vi "niRFUtil MT UTIL GenerateFilterCoefficients.vi"(9 "interpolation factor":i32=128, 10 "# of zero crossings":i32=16) -> (0 "full array size":i32, 1 "Differences (scaled)":T1 min=0 max=127 format="%.2f", 2 "Filter Coefficients (scaled)":T1 min=0 max=127 format="%.2f", 3 "Filter Coefficients (unscaled)":T1 min=0 max=127 format="%.2f")   [LabVIEW 2015, in "niRFUtil.lvlib"]
uses:
  niRFUtil.lvlib
  Includes/niRFUtil INC Real Array.ctl
  <vilib>/Analysis/4window.llb/windowTd.ctl
  <vilib>/Analysis/NI_AALBase.lvlib
  <vilib>/Analysis/NI_AALPro.lvlib
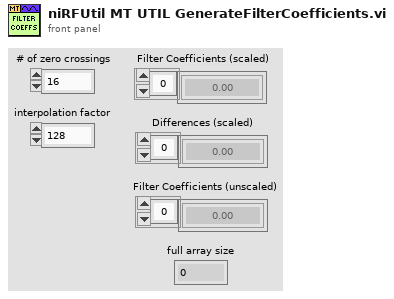
[diagram p1: front panel]
types:
  T1 = typedef "niRFUtil.lvlib/niRFUtil INC Real Array.ctl" = sgl[]
  T2 = typedef "NI_AALPro.lvlib/windowTd.ctl" = u32
  T3 = enum32{"Lowpass", "Highpass", "Bandpass", "Bandstop"}
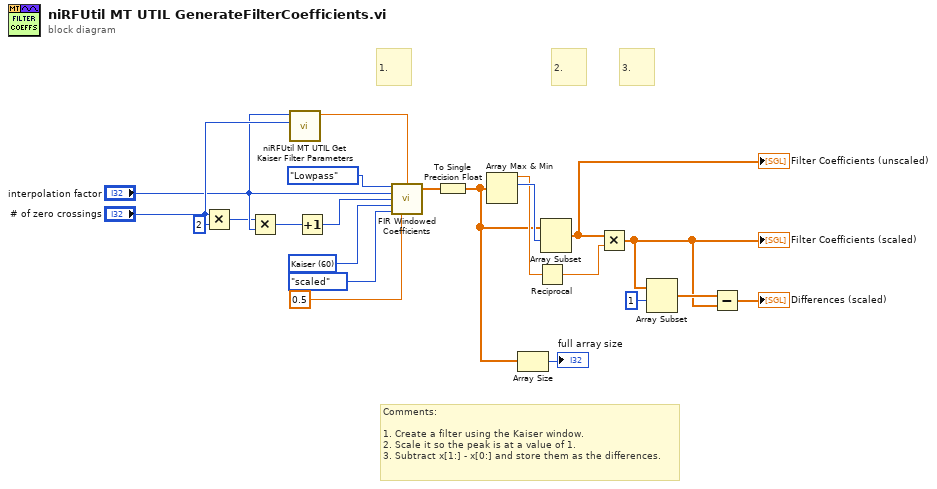
[diagram p0: block diagram]
diagram:
  w15 = T2 60 items=["Rectangle"=0, "Hanning"=1, "Hamming"=2, "Blackman-Harris"=3, "Exact Blackman"=4, "Blackman"=5, "Flat Top"=6, "4 Term B-Harris "=7, "7 Term B-Harris"=8, "Low Sidelobe"=9, "Blackman Nuttall"=11, "Triangle"=30, "Bartlett-Hanning"=31, "Bohman"=32, "Parzen"=33, "Welch"=34, "Kaiser"=60, "Dolph-Chebyshev"=61, "Gaussian"=62] ("window")
  # "Comments:\n\n1. Create a filter using the Kaiser window.\n2. Scale it so the peak is at a value of 1.\n3. Subtract x[1:] - x[0:] and store them as the differences."
  # "3."
  # "2."
  # "1."
  n1 = Multiply(x="# of zero crossings", y=2) -> (x*y=w7:i32)
  n2 = Multiply(x=w7, y="interpolation factor") -> (x*y=w8:i32)
  n3 = call "niRFUtil MT UTIL Get Kaiser Filter Parameters.vi"("len"="# of zero crossings", "I"="interpolation factor") -> ("beta"=w4:dbl)  [unwired: 2 in, 7 out]
  n4 = Increment(x=w8) -> (x+1=w5:i32)
  n5 = call <vilib>:"FIR Windowed Coefficients.vi"("filter type"=T3."Lowpass", "window parameter"=w4, "sampling freq: fs"="interpolation factor", "taps"=w5, "window"=w15, "option"=enum32{"not scaled", "scaled"}."scaled", "low cutoff freq: fl"=0.5) -> ("FIR Windowed Coefficients"=w10:dbl[])  [unwired: 1 in, 7 out]
  n6 = To Single Precision Float(number=w10) -> (single precision float=w1:sgl[])
  n7 = Array Max & Min(array=w1) -> (max value=w3:sgl, max index (indices)=w12:i32)  [unwired: 2 out]
  n8 = Array Size(array=w1) -> (size(s)=→"full array size":i32)
  n9 = Reciprocal(x=w3) -> (1/x=w2:sgl)
  n10 = Array Subset(array=w1, index=w12) -> (w22:sgl[])  [unwired: 1 in]
  "Filter Coefficients (unscaled)" <- w22
  n11 = Multiply(x=w22, y=w2) -> (x*y=w20:sgl[])
  "Filter Coefficients (scaled)" <- w20
  n12 = Array Subset(array=w20, index=1) -> (w21:sgl[])  [unwired: 1 in]
  n13 = Subtract(x=w21, y=w20) -> (x-y=→"Differences (scaled)":sgl[])
